vi "PQntuples.vi"(8 "error in (no error)":errorcluster, 10 "res":u32) -> (0 "error out":errorcluster, 1 "PQnTuples":i32, 2 "res out":u32)   [LabVIEW 2019, in "libpqlv.lvlib"]
doc: "Returns the number of rows (tuples) in the query result."
uses:
  libpqlv.lvlib
  libpq.dll
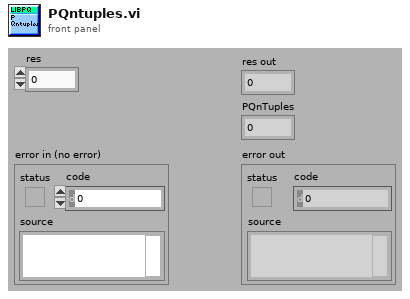
[diagram p1: front panel]
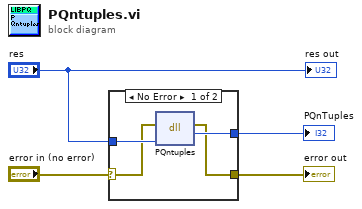
[diagram p0: block diagram]
diagram:
  n1 = case shown="No Error" "error in (no error)" {
    selector: "error in (no error)" -> [w6 w9]
    tunnel: [w5 w9] -> w3
    tunnel: "res" -> [w7 _]
    tunnel: [w8 _] -> w2
    frame No Error {
      n2 = dll-call lib="libpq.*" fn="PQntuples"(error in=w6, "res"=w7) -> (error out=w5:errorcluster, "PQnTuples"=w8:i32)  [unwired: 3 in, 1 out]
    }
    frame Error {
    }
  }
  "PQnTuples" <- w2
  "error out" <- w3
  "res out" <- "res"
